vi "Initialize.vi"(8 "error in (no error)":errorcluster, 10 "Laser Configuration":T1, 11 "Thorlabs Polarizer in":refnum<class "Thorlabs Polarizer.lvclass">) -> (0 "error out":errorcluster, 3 "Thorlabs Polarizer out":refnum<class "Thorlabs Polarizer.lvclass">)   [LabVIEW 2023, in "Thorlabs Polarizer.lvlib" / "Thorlabs Polarizer.lvclass"]
uses:
  Thorlabs Polarizer.lvclass
  Resources/Type Defs/Laser Configuration.ctl
  Thorlabs Polarizer.lvclass/Thorlabs Polarizer.ctl
  Thorlabs Polarizer.lvlib
  Laser/Laser.lvclass
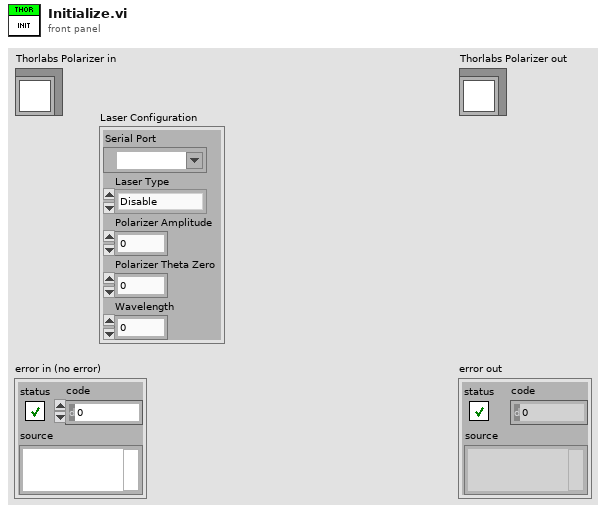
[diagram p1: front panel]
types:
  T1 = typedef "Laser Configuration.ctl" = cluster{"Serial Port":refnum<visa-resource-name>, "Laser Type":enum16{"Disable", "Laser Quantum", "Coherent OBIS", "PRM1-Z8", "Coherent HOPS"}, "Polarizer Amplitude":dbl, "Polarizer Theta Zero":dbl, "Wavelength":u16}
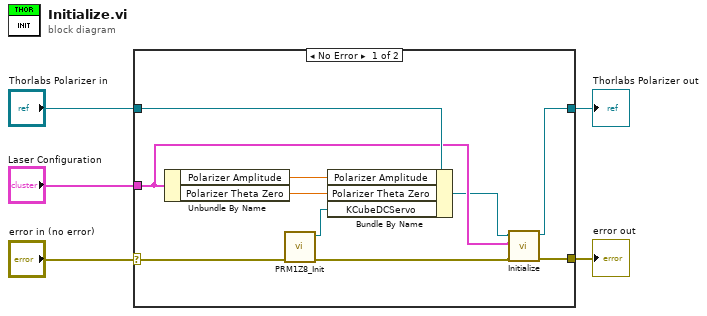
[diagram p0: block diagram]
diagram:
  n1 = case shown="No Error" "error in (no error)" {
    selector: "error in (no error)" -> [w15 w17]
    tunnel: [w6 w17] -> w4
    tunnel: [w7 w16] -> w2
    tunnel: "Thorlabs Polarizer in" -> [w14 w16]
    tunnel: "Laser Configuration" -> [w9 _]
    frame No Error {
      n2 = Unbundle By Name(w9) -> ("Polarizer Amplitude"=w12:dbl, "Polarizer Theta Zero"=w11:dbl)
      n3 = call "PRM1Z8_Init.vi"("error in (no error)"=w15) -> ("error out"=w10:errorcluster, "reference out"=w13:refnum<k24>)  [unwired: 9 in]
      n4 = Bundle By Name(cluster=w14, "Polarizer Amplitude"=w12, "Polarizer Theta Zero"=w11, "KCubeDCServo"=w13) -> (w8:refnum<class "Thorlabs Polarizer.lvclass">)
      n5 = call-parent "Initialize.vi"("error in (no error)"=w10, "Laser Configuration"=w9, "Laser in"=w8) -> ("error out"=w6:errorcluster, "Laser out"=w7:refnum<class "Thorlabs Polarizer.lvclass">)  [unwired: 7 in]
    }
    frame Error {
    }
  }
  "error out" <- w4
  "Thorlabs Polarizer out" <- w2
